vi "Get Item Attributes.vi"(10 "Item XLM String":string) -> (0 "URL":string, 1 "Type":string, 2 "Item Name":string)   [LabVIEW 2020, in "LV Project Items Parser.lvlib"]
doc: "Scans the XML item tag and returns the Name, Type, and URL attribute."
uses:
  LV Project Items Parser.lvlib
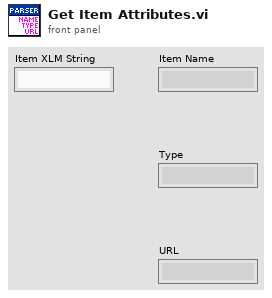
[diagram p1: front panel]
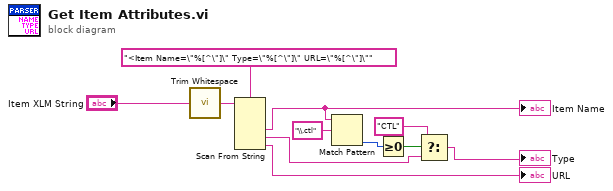
[diagram p0: block diagram]
diagram:
  n1 = call <vilib>:"Trim Whitespace.vi"("string"="Item XLM String") -> ("trimmed string"=w8:string)  [unwired: 1 in]
  n2 = Scan From String(format string="<Item Name=\"%[^\"]\" Type=\"%[^\"]\" URL=\"%[^\"]\"" ("String"), input string=w8) -> (output 1=w6:string, output 2=w3:string, output 3=→"URL":string)  [unwired: 5 in, 3 out]
  "Item Name" <- w6
  n3 = Match Pattern(string=w6, regular expression="\\.ctl") -> (offset past match=w4:i32)  [unwired: 1 in, 3 out]
  n4 = Greater Or Equal To 0?(x=w4) -> (x >= 0?=w5:bool)
  n5 = Select(t="CTL", s=w5, f=w3) -> (s? t:f=→"Type":string)
